vi "Query Calibration kits.vi"(8 "error in (no error)":errorcluster, 10 "Connector type":T1(ring), 11 "VNA-FieldFox in":refnum<class "VNA-FieldFox.lvclass">) -> (0 "error out":errorcluster, 2 "Cal kits instaled":string[](array[string]), 3 "VNA-FieldFox out":refnum<class "VNA-FieldFox.lvclass">)   [LabVIEW 2020, in "VNA-FieldFox.lvclass"]
doc: "Queryes the calibration kits installed on the VNA dependent on connector type.\nIf the VNA support E-cal it reports this aswell as the first sting in the array."
uses:
  VNA-FieldFox.lvclass
  Vector Network Analyzer.lvclass
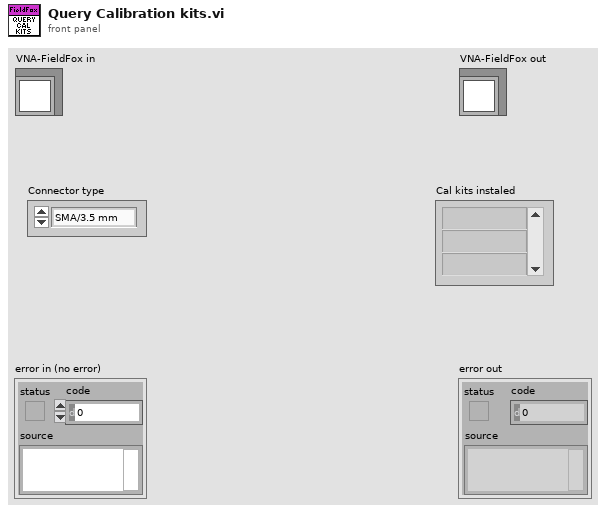
[diagram p1: front panel]
types:
  T1 = enum16{"SMA/3.5 mm", "2.92 mm", "2.4 mm", "1.85 mm", "N 50 Ohm", "N 75 Ohm", "7-16"}
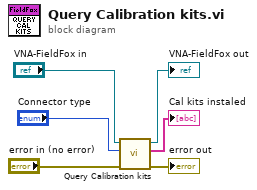
[diagram p0: block diagram]
diagram:
  n1 = call-parent "Query Calibration kits.vi"("error in (no error)"="error in (no error)", "Connector type"="Connector type", "Vector Network Analyzer in"="VNA-FieldFox in") -> ("error out"=→"error out":errorcluster, "Cal kits installed"=→"Cal kits instaled":string[], "Vector Network Analyzer out"=→"VNA-FieldFox out":refnum<class "VNA-FieldFox.lvclass">)  [unwired: 6 in]
